vi "CalibrationRead.vi"(0 "handle":u64, 3 "error in (no error)":errorcluster caption="错误输入（无错误）") -> (7 "handle out":u64, 8 "function return":i32, 9 "CalArray":u8[](array[numeric]), 10 "error out":errorcluster caption="错误输出")   [LabVIEW 2018]
doc: "Read Calibration Config Array from the device's EEPROM."
uses:
  InstrumentsPlayground.lvlib
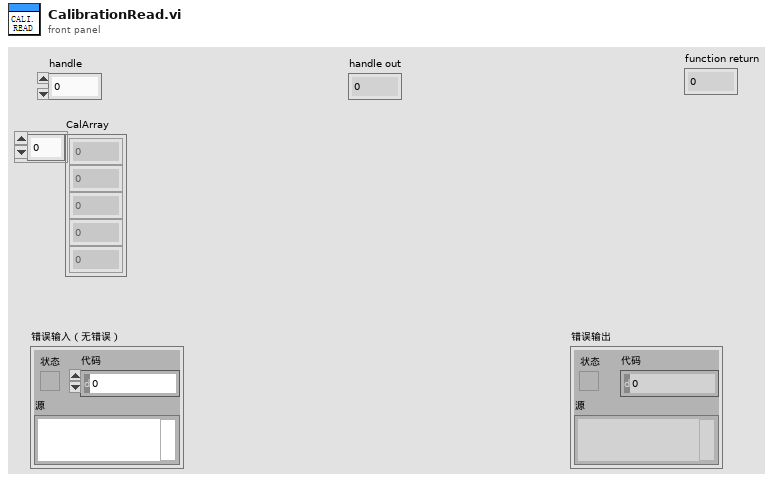
[diagram p1: front panel]
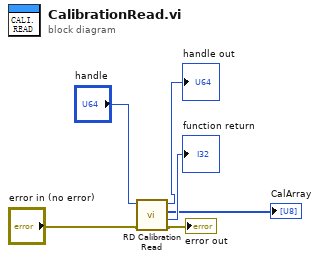
[diagram p0: block diagram]
diagram:
  n1 = call "RD Calibration Read.vi"("error in (no error)"="error in (no error)", "handle"="handle") -> ("error out"=→"error out":errorcluster, "function return"=→"function return":i32, "CalArray out"=→"CalArray":u8[], "handle out"=→"handle out":u64)  [unwired: 6 in]
